vi "ifr2025 RF Limit.vi"(7 "Limit (Enable)":bool=TRUE, 8 "error in (no error)":errorcluster {"code" format="%.0x"}, 9 "Unit (dBm)":i16(ring) items=["dBm", "dBV", "dBmV", "dBuV", "V", "mV", "uV"], 10 "Level (19.0)":dbl=19.0, 11 "instrument handle":refnum<visa-resource-name>) -> (0 "error out":errorcluster {"code" format="%.0x"}, 3 "instrument handle out":refnum<visa-resource-name>)   [LabVIEW 2009]
doc: "Allows the RF output to be assigned a user programmed limit."
uses:
  Ifr2025_32.dll
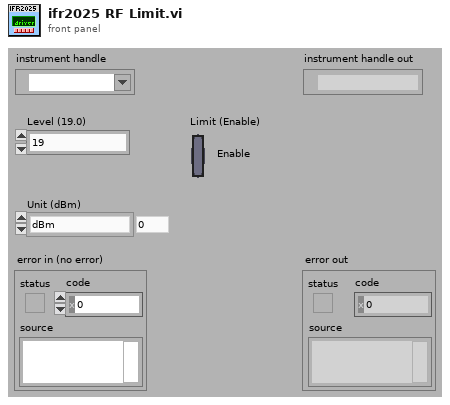
[diagram p1: front panel]
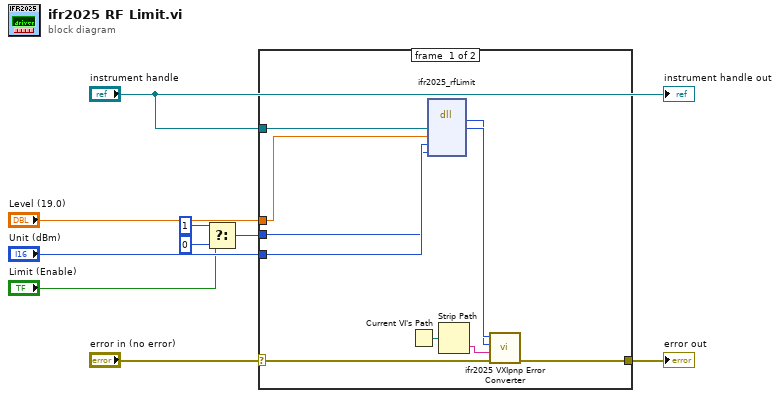
[diagram p0: block diagram]
diagram:
  n1 = Select(t=i16 1, s="Limit (Enable)", f=i16 0) -> (s? t:f=w1:i16)
  n2 = case shown="No Error" "error in (no error)" {
    selector: "error in (no error)" -> [w14 w20]
    tunnel: [w13 w20] -> w9
    tunnel: "instrument handle" -> [w18 _]
    tunnel: "Level (19.0)" -> [w12 _]
    tunnel: "Unit (dBm)" -> [w11 _]
    tunnel: w1 -> [w10 _]
    frame #0 {
      n3 = Current VI's Path() -> (path=w19:path)
      n4 = dll-call lib="P:/inst/Marconi 2024 Signal Generator/source/labview/ifr2025/ifr2025/ifr2025_*.*" fn="ifr2025_rfLimit"("vi"=w18, "Level"=w12, "Unit"=w11, "Limit"=w10) -> (w16:i32, "vi"=w17:u32)  [unwired: 6 in, 2 out]
      n5 = Strip Path(path=w19) -> (name=w15:string)  [unwired: 1 out]
      n6 = call "ifr2025 VXIpnp Error Converter.vi"("error in (no error)"=w14, "name of VI (\"\")"=w15, "CVI error code (0)"=w16, "instrument handle"=w17) -> ("error out"=w13:errorcluster)  [unwired: 7 out]
    }
    frame #1 {
    }
  }
  "error out" <- w9
  "instrument handle out" <- "instrument handle"
